vi "mult_process_premade.vi"() -> ()   [LabVIEW 2013]
uses:
  results_cluster.ctl
  <vilib>/Utility/file.llb/Read From Spreadsheet File (DBL).vi
  <vilib>/gmath/statdist.llb/Student t Inverse CDF.vi
  <vilib>/Analysis/NI_AALBase.lvlib
  <vilib>/gmath/NI_Gmath.lvlib
panel:
  out "Промахи":bool
  in  "Уровень значимости":dbl
  in  "Критерий Граббса":bool
  in  "Строка форматирования":string="%_5f ± %_3f; %_2f"
  out "Результат измерений":string
  in  "Pдов":dbl=0.95
  in  "Границы НСП":dbl
  out "Результаты обработки":T1 {"Dдов рез" format="%#.4g"; "S сумм" format="%#.4g"; "К" format="%#.4g"; "Dдов случ." format="%#.4g"; "Sхср" format="%#.4g"; "S" format="%#.4g"}
  in  "Записать результат":bool
  in  "Получить данные":bool
  in  "Вычислить Dдов":bool
  out "Ряд измерений":dbl[](graph)
  in  "Стоп":bool
  in  "Вычислить оценки":bool
  in  "Путь":path caption="Путь к файлу"
  # "Обработка результатов многократных измерений"
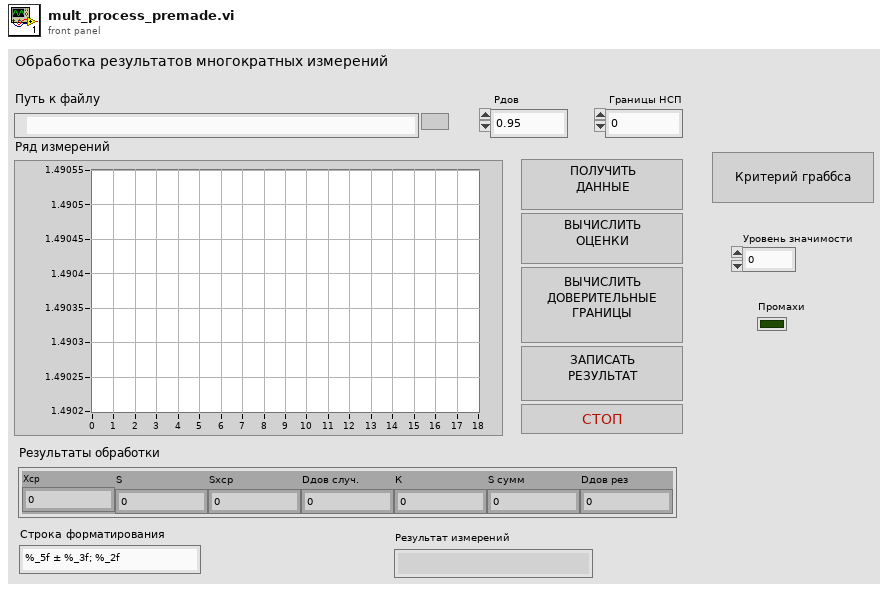
[diagram p1: front panel]
types:
  T1 = typedef "results_cluster.ctl" = cluster{"Xср":dbl, "S":dbl, "Sхср":dbl, "Dдов случ.":dbl, "К":dbl, "S сумм":dbl, "Dдов рез":dbl}
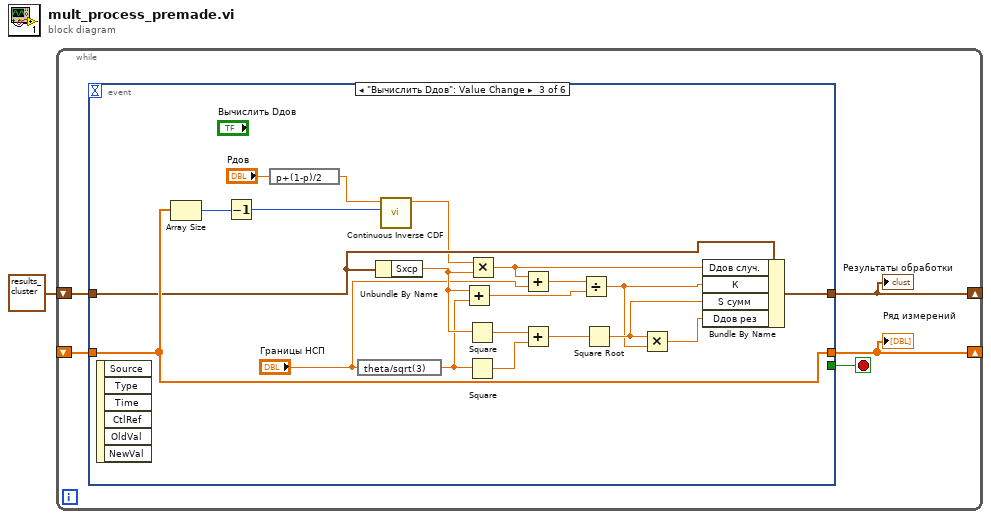
[diagram p0: block diagram]
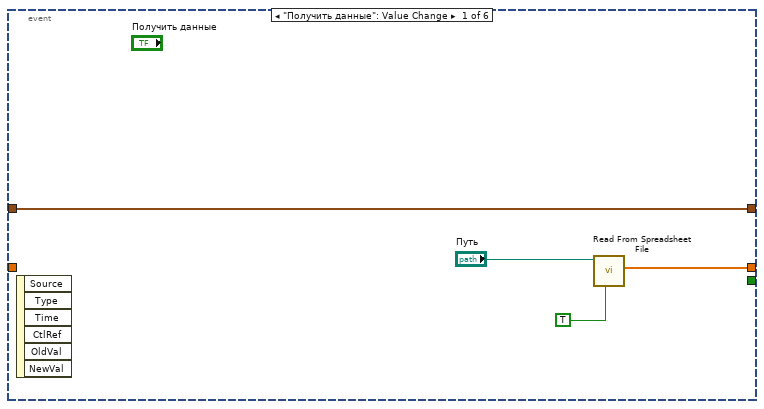
[diagram p2: hidden frame]
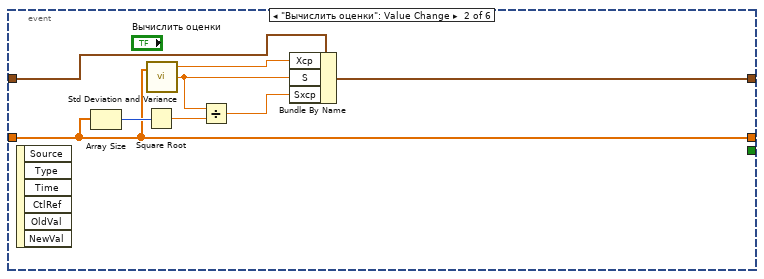
[diagram p3: hidden frame]
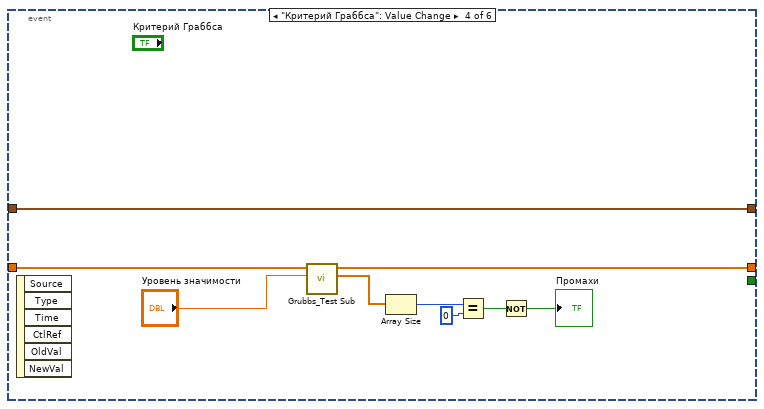
[diagram p4: hidden frame]
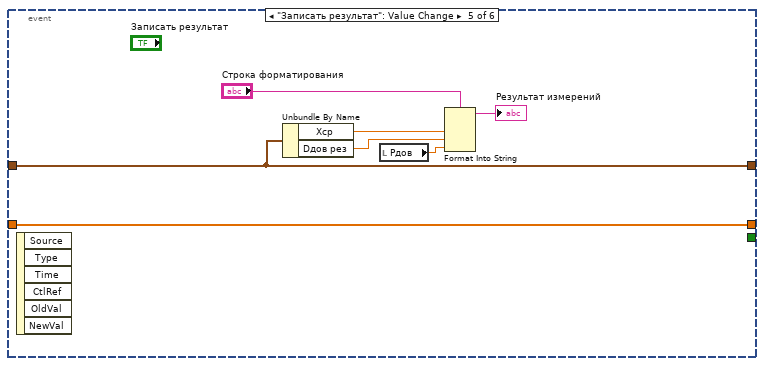
[diagram p5: hidden frame]
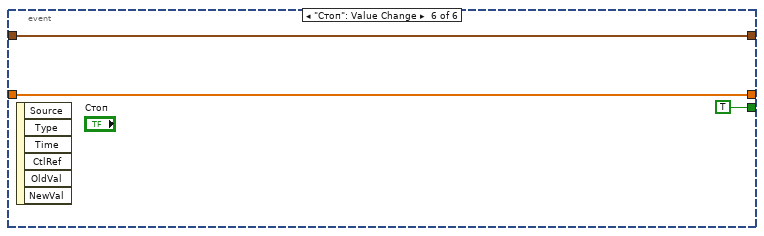
[diagram p6: hidden frame]
diagram:
  n1 = while {
    shift-right: [w4] -> _
    shift-left: _ -> [w5]
    shift-right: [w3] -> _
    shift-left: T1 {"Xср"=1.3199999999999998, "S"=0.130384048104053, "Sхср"=0.05830951894845301, "Dдов случ."=0.16189317847087023, "К"=2.43060784036949, "S сумм"=0.06506407098647712, "Dдов рез"=0.15814524106608838} ("Результаты обработки") -> [w6]
    stop <- w2 stop-if-true
    n2 = event shown="[2] \"Вычислить Dдов\": Value Change" {
      selector: _ -> [_ _ _ _ _ _]
      dyn-events: _ -> [_ _ _ _ _ _]
      timeout: _ -> [_ _ _ _ _ _]
      tunnel: [w8 w11 w34 w47 w53 w56] -> w4
      tunnel: w6 -> [w7 w18 w27 w39 w54 w57]
      tunnel: [w7 w17 w28 w39 w54 w57] -> w3
      tunnel: w5 -> [_ w11 w34 w46 w53 w56]
      tunnel: [_ _ _ _ _ TRUE] -> w2
      event "Получить данные": Value Change {
        n3 = event-data() -> ()  [unwired: 1 in, 6 out]
        n4 = call-poly <vilib>:"Read From Spreadsheet File.vi"("transpose (no:F)"=TRUE, "file path (dialog if empty)"="Путь") -> ("first row"=w8:dbl[])  [unwired: 5 in, 4 out]
      }
      event "Вычислить оценки": Value Change {
        n5 = event-data() -> ()  [unwired: 1 in, 6 out]
        n6 = Array Size(array=w11) -> (size(s)=w15:i32)
        n7 = Square Root(x=w15) -> (sqrt(x)=w13:dbl)
        n8 = call <vilib>:"Std Deviation and Variance.vi"("X"=w11) -> ("mean"=w16:dbl, "standard deviation"=w14:dbl)  [unwired: 1 in, 1 out]
        n9 = Divide(x=w14, y=w13) -> (x/y=w12:dbl)
        n10 = Bundle By Name(cluster=w18, "Xср"=w16, "S"=w14, "Sхср"=w12) -> (w17:T1)
      }
      event "Вычислить Dдов": Value Change {
        n11 = event-data() -> ()  [unwired: 1 in, 6 out]
        n12 = Array Size(array=w34) -> (size(s)=w36:i32)
        n13 = Decrement(x=w36) -> (x-1=w35:i32)
        n14 = expression code="p+(1-p)/2"("Pдов") -> (w37:dbl)
        n15 = expression code="theta/sqrt(3)"("Границы НСП") -> (w21:dbl)
        n16 = Unbundle By Name(w27) -> ("Sхср"=w22:dbl)
        n17 = call-poly <vilib>:"Continuous Inverse CDF.vi"("k degrees of freedom"=w35, "cdf(x)"=w37) -> ("x"=w23:dbl)  [unwired: 8 in, 1 out]
        n18 = Add(x=w22, y=w21) -> (x+y=w29:dbl)
        n19 = Square(x=w22) -> (x^2=w32:dbl)
        n20 = Square(x=w21) -> (x^2=w33:dbl)
        n21 = Multiply(x=w23, y=w22) -> (x*y=w19:dbl)
        n22 = Add(x=w19, y="Границы НСП") -> (x+y=w30:dbl)
        n23 = Add(x=w32, y=w33) -> (x+y=w31:dbl)
        n24 = Divide(x=w30, y=w29) -> (x/y=w24:dbl)
        n25 = Square Root(x=w31) -> (sqrt(x)=w25:dbl)
        n26 = Multiply(x=w25, y=w24) -> (x*y=w26:dbl)
        n27 = Bundle By Name(cluster=w27, "Dдов случ."=w19, "К"=w24, "S сумм"=w25, "Dдов рез"=w26) -> (w28:T1)
      }
      event "Критерий Граббса": Value Change {
        n28 = event-data() -> ()  [unwired: 1 in, 6 out]
        n29 = call "Grubbs_Test Sub.vi"("Уровень значимости"="Уровень значимости", "Исходная выборка"=w46) -> ("Array"=w44:dbl[], "Обработанные результаты"=w47:dbl[])  [unwired: 2 in, 2 out]
        n30 = Array Size(array=w44) -> (size(s)=w43:i32)
        n31 = Equal?(x=w43, y=0) -> (x = y?=w42:bool)
        n32 = Not(x=w42) -> (.not. x?=→"Промахи":bool)
      }
      event "Записать результат": Value Change {
        n33 = event-data() -> ()  [unwired: 1 in, 6 out]
        n34 = Unbundle By Name(w54) -> ("Xср"=w50:dbl, "Dдов рез"=w51:dbl)
        n35 = local read "Pдов"() -> (w52:dbl)
        n36 = Format Into String(format string="Строка форматирования", w50, w51, w52) -> (resulting string=→"Результат измерений":string)  [unwired: 2 in, 1 out]
      }
      event "Стоп": Value Change {
        n37 = event-data() -> ()  [unwired: 1 in, 6 out]
      }
    }
    "Ряд измерений" <- w4
    "Результаты обработки" <- w3
  }
